vi "Test MainUI API.vi"() -> ()   [LabVIEW 2020]
doc: "CML UI API Tester.\n_____\nBased on Delacor QMH Project Template 5.0.0.82."
uses:
  MainUI.lvlib
panel:
  out "error out":errorcluster
  in  "Show Block Diagram":bool
  in  "Stop Module":bool
  in  "Start Module":bool
  in  "Hide Module Panel":bool
  in  "Show Module Panel":bool
  out "Status":string
  out "Module Running?":bool
  # "This VI tests the API for the Module."
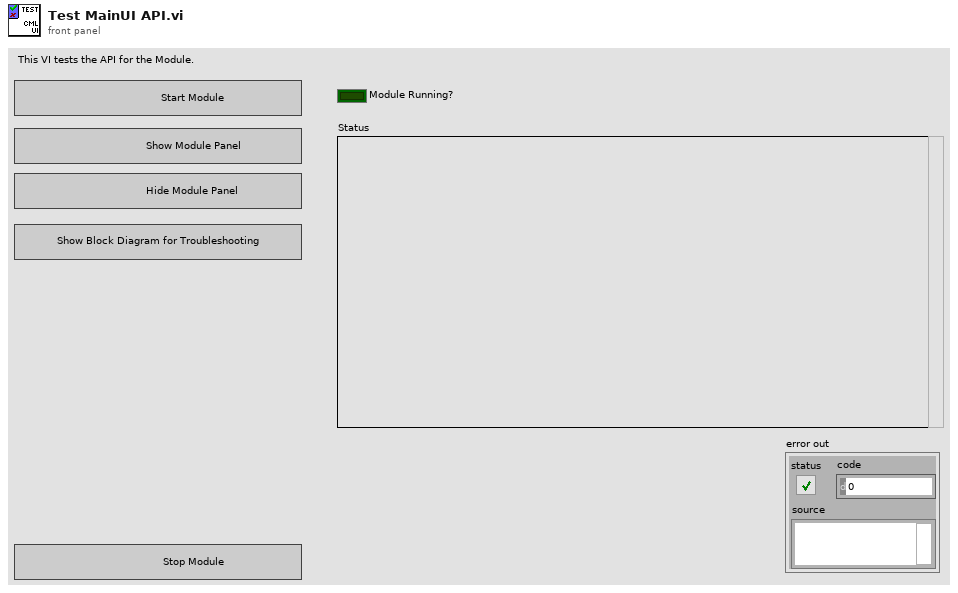
[diagram p1: front panel]
types:
  T1 = typedef "MainUI.lvlib/Broadcast Events--cluster.ctl" = cluster{"Module Did Init":refnum<user-event>, "Status Updated":refnum<user-event>, "Error Reported":refnum<user-event>, "Module Did Stop":refnum<user-event>, "Update Module Execution Status":refnum<user-event>}
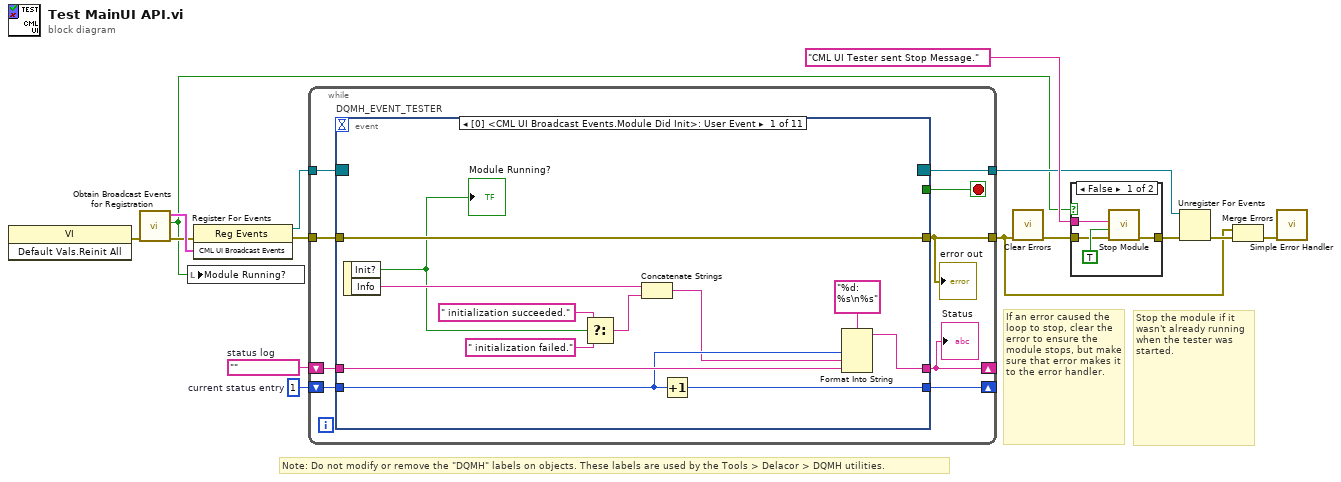
[diagram p0: block diagram]
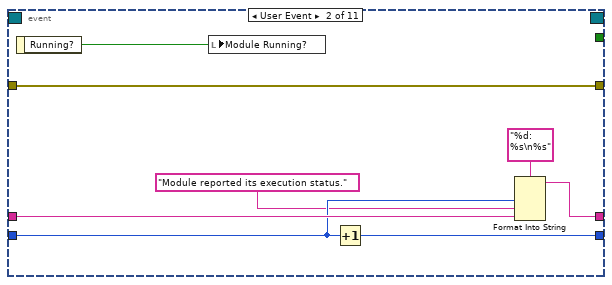
[diagram p3: hidden frame]
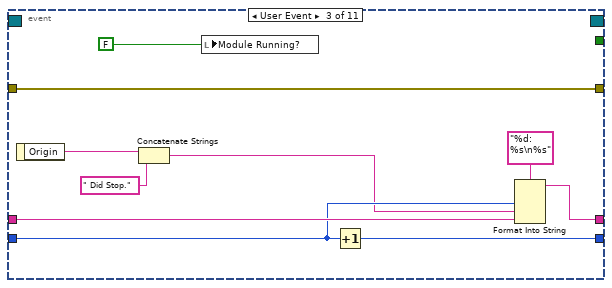
[diagram p4: hidden frame]
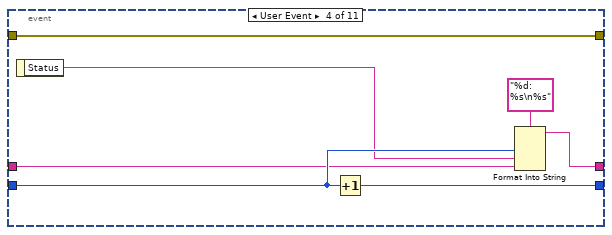
[diagram p5: hidden frame]
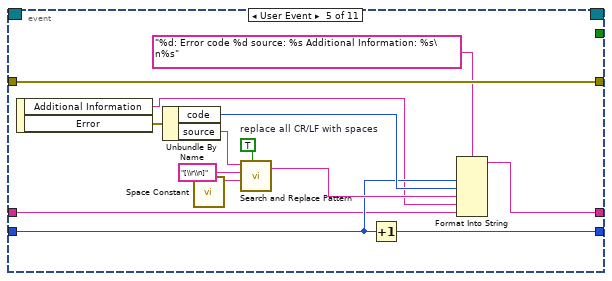
[diagram p6: hidden frame]
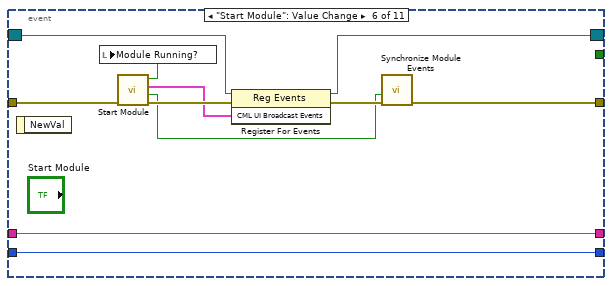
[diagram p7: hidden frame]
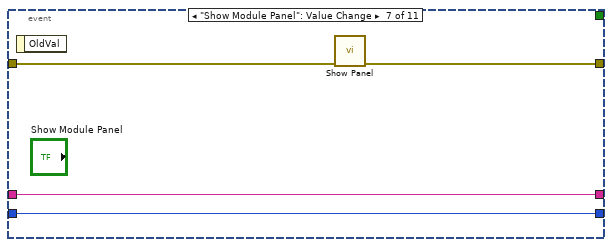
[diagram p8: hidden frame]
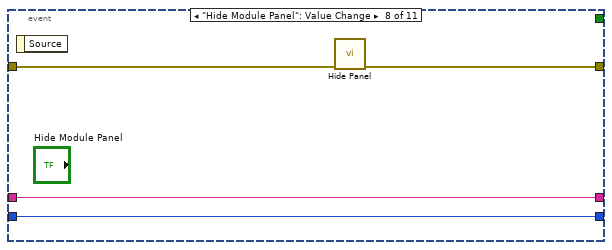
[diagram p9: hidden frame]
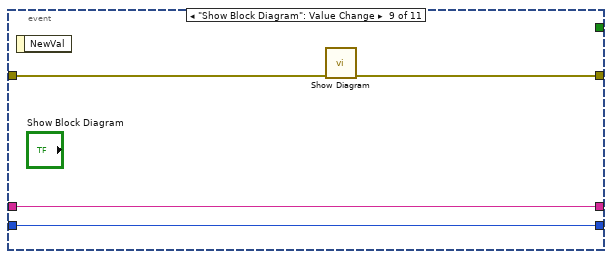
[diagram p10: hidden frame]
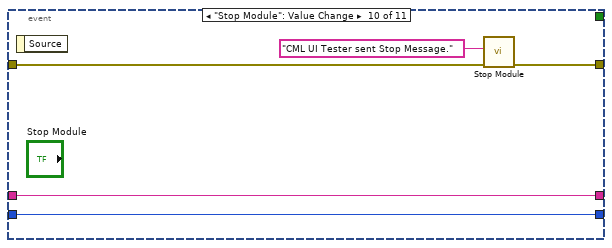
[diagram p11: hidden frame]
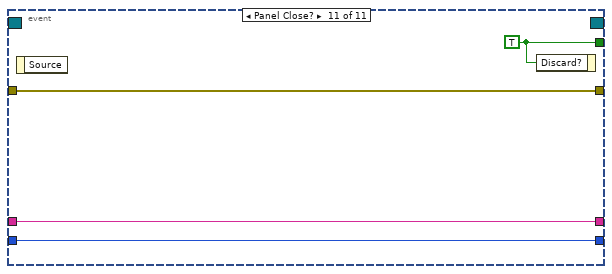
[diagram p12: hidden frame]
diagram:
  w11 = 1  # current status entry
  w12 = ""  # status log
  # "Stop the module if it wasn't already running when the tester was started."
  # "If an error caused the loop to stop, clear the error to ensure the module stops, but make sure that error makes it to the error handler."
  # "Note: Do not modify or remove the \"DQMH\" labels on objects. These labels are used by the Tools > Delacor > DQMH utilities."
  n1 = invoke class="VI" method="Default Vals.Reinit All"() -> (error out=w3:errorcluster)  [unwired: 3 in, 2 out]
  n2 = call "Obtain Broadcast Events for Registration.vi"("error in (no error)"=w3) -> ("error out"=w2:errorcluster, "Already running?"=w1:bool, "CML UI Broadcast Events"=w9:T1)  [unwired: 8 in]
  n3 = local write "Module Running?"(w1) -> ()
  n4 = register-events(error in=w2, w9) -> (reference out=w8:refnum<event-registration>, error out=w10:errorcluster)  [unwired: 1 in]
  n5 = while {
    tunnel: w8 -> [w24]
    tunnel: [w17] -> w4
    shift-right: [w20] -> _
    shift-left: w12 -> [w22]
    shift-right: [w21] -> _
    shift-left: w11 -> [w23]
    tunnel: w10 -> [w19]
    tunnel: [w18] -> w7
    stop <- w16 stop-if-true
    n6 = event "DQMH_EVENT_TESTER" shown="[0] <CML UI Broadcast Events.Module Did Init>: User Event" {
      selector: w24 -> [_ _ _ _ _ w80 _ _ _ _ _]
      dyn-events: [_ _ _ _ _ w79 _ _ _ _ _] -> w18
      timeout: _ -> [_ _ _ _ _ _ _ _ _ _ _]
      tunnel: [_ _ _ _ _ _ _ _ _ _ w107] -> w16
      tunnel: [w36 w38 w45 w55 w75 w78 w90 w94 w95 w101 w104] -> w17
      tunnel: w23 -> [w33 w42 w52 w58 w65 w83 w88 w92 w96 w102 w105]
      tunnel: w22 -> [w34 w43 w53 w57 w63 w84 w89 w93 w97 w103 w106]
      tunnel: [w31 w40 w50 w59 w66 w84 w89 w93 w97 w103 w106] -> w20
      tunnel: [w32 w41 w51 w61 w64 w83 w88 w92 w96 w102 w105] -> w21
      tunnel: w19 -> [w36 w38 w45 w55 w75 w77 w87 w91 w98 w99 w104]
      event User Event {
        n7 = event-data() -> ("Init?"=w28:bool, "Info"=w30:string)  [unwired: 1 in]
        "Module Running?" <- w28
        n8 = Select(t=" initialization succeeded.", s=w28, f=" initialization failed.") -> (s? t:f=w25:string)
        n9 = Concatenate Strings(w30, w25) -> (w29:string)
        n10 = Increment(x=w33) -> (x+1=w32:i32)
        n11 = Format Into String(format string="%d: %s\n%s", w33, w29, w34) -> (resulting string=w31:string)  [unwired: 2 in, 1 out]
      }
      event User Event {
        n12 = event-data() -> ("Running?"=w37:bool)  [unwired: 1 in]
        n13 = local write "Module Running?"(w37) -> ()
        n14 = Increment(x=w42) -> (x+1=w41:i32)
        n15 = Format Into String(format string="%d: %s\n%s", w42, "Module reported its execution status.", w43) -> (resulting string=w40:string)  [unwired: 2 in, 1 out]
      }
      event User Event {
        n16 = event-data() -> ("Origin"=w49:string)  [unwired: 1 in]
        n17 = Concatenate Strings(w49, " Did Stop.") -> (w48:string)
        n18 = local write "Module Running?"(FALSE ("Module Did Init?")) -> ()
        n19 = Increment(x=w52) -> (x+1=w51:i32)
        n20 = Format Into String(format string="%d: %s\n%s", w52, w48, w53) -> (resulting string=w50:string)  [unwired: 2 in, 1 out]
      }
      event User Event {
        n21 = event-data() -> ("Status"=w56:string)  [unwired: 1 in]
        n22 = Increment(x=w58) -> (x+1=w61:i32)
        n23 = Format Into String(format string="%d: %s\n%s", w58, w56, w57) -> (resulting string=w59:string)  [unwired: 2 in, 1 out]
      }
      event User Event {
        w71 = TRUE  # replace all CR/LF with spaces
        n24 = event-data() -> ("Additional Information"=w62:string, "Error"=w67:errorcluster)  [unwired: 1 in]
        n25 = Unbundle By Name(w67) -> ("code"=w68:i32, "source"=w69:string)
        n26 = call <vilib>:"Space Constant.vi"() -> ("String"=w72:string)
        n27 = call <vilib>:"Search and Replace Pattern.vi"("string"=w69, "regular expression (\"\")"="[\\r\\n]" ("regular expression (\"\")"), "replace string (\"\")"=w72, "replace all? (F)"=w71) -> ("result string"=w70:string)  [unwired: 1 in, 1 out]
        n28 = Increment(x=w65) -> (x+1=w64:i32)
        n29 = Format Into String(format string="%d: Error code %d source: %s Additional Information: %s\n%s", w65, w68, w70, w62, w63) -> (resulting string=w66:string)  [unwired: 2 in, 1 out]
      }
      event "Start Module": Value Change {
        n30 = event-data() -> ()  [unwired: 1 in, 1 out]
        n31 = call "Start Module.vi"("error in (no error)"=w77) -> ("error out"=w85:errorcluster, "Wait for Event Sync?"=w82:bool, "CML UI Broadcast Events"=w81:T1, "Module Was Already Running?"=w76:bool)  [unwired: 7 in]
        n32 = local write "Module Running?"(w76) -> ()
        n33 = register-events(reference=w80, error in=w85, w81) -> (reference out=w79:refnum<event-registration>, error out=w86:errorcluster)
        n34 = call "Synchronize Module Events.vi"("error in (no error)"=w86, "Wait for Event Sync?"=w82) -> ("error out"=w78:errorcluster)  [unwired: 9 in]
      }
      event "Show Module Panel": Value Change {
        n35 = event-data() -> ()  [unwired: 1 in, 1 out]
        n36 = call "Show Panel.vi"("error in (no error)"=w87) -> ("error out"=w90:errorcluster)  [unwired: 10 in]
      }
      event "Hide Module Panel": Value Change {
        n37 = event-data() -> ()  [unwired: 1 in, 1 out]
        n38 = call "Hide Panel.vi"("error in (no error)"=w91) -> ("error out"=w94:errorcluster)  [unwired: 10 in]
      }
      event "Show Block Diagram": Value Change {
        n39 = event-data() -> ()  [unwired: 1 in, 1 out]
        n40 = call "Show Diagram.vi"("error in (no error)"=w98) -> ("error out"=w95:errorcluster)  [unwired: 10 in]
      }
      event "Stop Module": Value Change {
        n41 = event-data() -> ()  [unwired: 1 in, 1 out]
        n42 = call "Stop Module.vi"("error in (no error)"=w99, "Origin"="CML UI Tester sent Stop Message.") -> ("error out"=w101:errorcluster)  [unwired: 9 in]
      }
      event Panel Close? {
        w107 = TRUE ("Discard?")
        n43 = event-data() -> ()  [unwired: 1 in, 1 out]
        n44 = event-data("Discard?"=w107) -> ()  [unwired: 1 in, 1 out]
      }
    }
    "Status" <- w20
    "error out" <- w17
  }
  n45 = call <vilib>:"Clear Errors.vi"("error in (no error)"=w4) -> ("error out"=w6:errorcluster)  [unwired: 5 in, 1 out]
  n46 = case shown="False" w1 {
    tunnel: [w111 w112] -> w14
    tunnel: "CML UI Tester sent Stop Message." ("Origin") -> [w110 _]
    tunnel: w6 -> [w108 w112]
    frame False {
      n47 = call "Stop Module.vi"("error in (no error)"=w108, "Wait for Module to Stop? (F)"=TRUE ("Wait for Module to stop?"), "Origin"=w110) -> ("error out"=w111:errorcluster)  [unwired: 8 in]
    }
    frame True {
    }
  }
  n48 = Unregister For Events(event registration refnum=w7, error in=w14) -> (error out=w15:errorcluster)
  n49 = Merge Errors(w4, w15) -> (w5:errorcluster)
  n50 = call <vilib>:"Simple Error Handler.vi"("error in (no error)"=w5) -> ()  [unwired: 4 in, 5 out]
